vi "AguaClara Server Test.vi"() -> ()   [LabVIEW 2015, in "AguaClara Library.lvlib"]
uses:
  AguaClara Library.lvlib
  mathcad/Simple/MathCAD cmd.ctl
  <vilib>/Utility/SMTP/NI_SMTPEmail.lvlib
  Word cmd.ctl
  Variable cluster.ctl
  User Information.ctl
  Project inputs.ctl
  Basic Inputs.ctl
  user project design.ctl
  ADT Commands.ctl
  Country Ring.ctl
panel:
  in  "reload MathCAD":bool
  out "total requests":i32
  in  "ADT version":i32
  out "Revision":i32
  in  "SVN Checkout":bool
  in  "Progress bar":dbl(slide) max=314.0 scale=0.0..1.0
  out "DesignLog":refnum<file>
  out "Designs in queue":i32
  out "Loaded CAD":bool
  in  "File Directories":bool
  in  "millisecond multiple":u32=100
  out "stop loops":bool
  in  "stop":bool
  in  "Tab Control":T1(tab)=enum."Test Design"
  out "User Project Design":T2[](array[typedef])
  out "MathCAD Results":T3
  out "Find-Replace":cluster{"Find":string, "Replace":string}[](array[cluster])
  in  "Load Client Design":i32
  in  "Design Inputs":T4={"Q.Plant"=0.005, "C.CoagDoseMax"=0.1, "C.CoagStock"=120.0, "Ti.CoagStock"=108000.0, "EN.DrillSeries"=enum."English", "EN.TubeSeries"=enum."English", "N.SedTanks"=8.0, "N.SedBaysEst"=2.0, "W.SedPlate"=0.01, "L.SedPlateSheet"=1.08, "T.SedPlate"=3.0, "T.PlantWall"=0.002, "H.FlocOption"=0.15, "T.FlocBaffleRigidH"=1.0, "T.ConcreteMin"=0.04, "T.SedWeir"=0.05, "T.FlocBaffleRigidV"=0.05} caption="Basic Inputs" {"T.FlocBaffleRigidV" min=0.0 max=0.2 step=0.001 format="%#.1f"; "T.SedWeir" min=0.001 max=0.2 step=0.001 format="%#.1f"; "T.SedPlate" min=0.001 max=0.05 step=0.001 format="%#.1f"; "T.FlocBaffleRigidH" min=0.0 max=0.2 step=0.001 format="%#.1f"; "T.ConcreteMin" min=0.005 max=0.2 step=0.001 format="%#.1f"; "L.SedPlateSheet" min=0.3 max=8.0 step=0.01 format="%#.1f"; "N.SedBaysEst" min=1.0 max=20.0 step=1.0 format="%#.0f"; "N.SedTanks" min=1.0 max=20.0 step=1.0 format="%#.0f"; "Ti.CoagStock" min=43200.0 max=360000.0 step=3600.0 format="%#.1f"; "H.FlocOption" min=0.5 max=4.0 step=0.01 format="%#.2f"; "C.CoagStock" min=50.0 max=500.0 step=1.0 format="%#.0f"; "C.CoagDoseMax" min=0.03 max=0.2 step=0.005 format="%#.0f"; "Q.Plant" min=0.001 max=0.2 step=0.0001 format="%#.1f"; "T.PlantWall" min=0.05 max=0.5 step=0.001 format="%#.1f"; "W.SedPlate" min=0.5 max=3.0 step=0.001 format="%#.1f"}
  in  "Project Info":T5={"Project Name"="ADT Server Test", "City"="Ithaca", "State"="NY", "Notes"="USA"} caption="Project Information"
  in  "User Information":T6={"First Name"="Agua", "Last Name"="Clara", "Email Address"="cuaguaclara@gmail.com", "Organization"="Cornell University", "Language"=enum."English", "Country"=0} {"Country" items=["Afghanistan", "Aland Islands", "Albania", "Algeria", "American Samoa", "Andorra", "Angola", "Anguilla", "Antarctica", "Antigua And Barbuda", "Argentina", "Armenia", "Aruba", "Australia", "Austria", "Azerbaijan", "Bahamas", "Bahrain", "Bangladesh", "Barbados", "Belarus", "Belgium", "Belize", "Benin", "Bermuda", "Bhutan", "Bolivia", "Bosnia And Herzegovina", "Botswana", "Bouvet Island", "Brazil", "British Indian Ocean Territory", "Brunei Darussalam", "Bulgaria", "Burkina Faso", "Burundi", "Cambodia", "Cameroon", "Canada", "Cape Verde", "Cayman Islands", "Central African Republic", "Chad", "Chile", "China", "Christmas Island", "Cocos (Keeling) Islands", "Colombia", "Comoros", "Congo", "Congo, The Democratic Republic Of The", "Cook Islands", "Costa Rica", "Cote D'Ivoire", "Croatia", "Cuba", "Cyprus", "Czech Republic", "Denmark", "Djibouti", "Dominica", "Dominican Republic", "Ecuador", "Egypt", "El Salvador", "Equatorial Guinea", "Eritrea", "Estonia", "Ethiopia", "Falkland Islands (Malvinas)", "Faroe Islands", "Fiji", "Finland", "France", "French Guiana", "French Polynesia", "French Southern Territories", "Gabon", "Gambia", "Georgia", "Germany", "Ghana", "Gibraltar", "Greece", "Greenland", "Grenada", "Guadeloupe", "Guam", "Guatemala", "Guernsey", "Guinea", "Guinea-Bissau", "Guyana", "Haiti", "Heard Island And Mcdonald Islands", "Holy See (Vatican City State)", "Honduras", "Hong Kong", "Hungary", "Iceland", "India", "Indonesia", "Iran, Islamic Republic Of", "Iraq", "Ireland", "Isle Of Man", "Israel", "Italy", "Jamaica", "Japan", "Jersey", "Jordan", "Kazakhstan", "Kenya", "Kiribati", "Korea, Democratic People'S Republic Of", "Korea, Republic Of", "Kuwait", "Kyrgyzstan", "Lao People'S Democratic Republic", "Latvia", "Lebanon", "Lesotho", "Liberia", "Libyan Arab Jamahiriya", "Liechtenstein", "Lithuania", "Luxembourg", "Macao", "Macedonia, The Former Yugoslav Republic Of", "Madagascar", "Malawi", "Malaysia", "Maldives", "Mali", "Malta", "Marshall Islands", "Martinique", "Mauritania", "Mauritius", "Mayotte", "Mexico", "Micronesia, Federated States Of", "Moldova, Republic Of", "Monaco", "Mongolia", "Montserrat", "Morocco", "Mozambique", "Myanmar", "Namibia", "Nauru", "Nepal", "Netherlands", "Netherlands Antilles", "New Caledonia", "New Zealand", "Nicaragua", "Niger", "Nigeria", "Niue", "Norfolk Island", "Northern Mariana Islands", "Norway", "Oman", "Pakistan", "Palau", "Palestinian Territory, Occupied", "Panama", "Papua New Guinea", "Paraguay", "Peru", "Philippines", "Pitcairn", "Poland", "Portugal", "Puerto Rico", "Qatar", "Reunion", "Romania", "Russian Federation", "Rwanda", "Saint Helena", "Saint Kitts And Nevis", "Saint Lucia", "Saint Pierre And Miquelon", "Saint Vincent And The Grenadines", "Samoa", "San Marino", "Sao Tome And Principe", "Saudi Arabia", "Senegal", "Serbia And Montenegro", "Seychelles", "Sierra Leone", "Singapore", "Slovakia", "Slovenia", "Solomon Islands", "Somalia", "South Africa", "South Georgia And The South Sandwich Islands", "Spain", "Sri Lanka", "Sudan", "Suriname", "Svalbard And Jan Mayen", "Swaziland", "Sweden", "Switzerland", "Syrian Arab Republic", "Taiwan, Province Of China", "Tajikistan", "Tanzania, United Republic Of", "Thailand", "Timor-Leste", "Togo", "Tokelau", "Tonga", "Trinidad And Tobago", "Tunisia", "Turkey", "Turkmenistan", "Turks And Caicos Islands", "Tuvalu", "Uganda", "Ukraine", "United Arab Emirates", "United Kingdom", "United States", "United States Minor Outlying Islands", "Uruguay", "Uzbekistan", "Vanuatu", "Venezuela", "Viet Nam", "Virgin Islands, British", "Virgin Islands, U.S.", "Wallis And Futuna", "Western Sahara", "Yemen", "Zambia", "Zimbabwe", "(Not Specified)"]}
  in  "Recreate Design":bool
  out "Date":string
  out "Last Design":i32
  out "init errors":errorcluster caption="error out"
  out "commandline":string
  out "SVN Checkout output":string
  out "design errors":errorcluster
  out "error out design log":errorcluster
  out "ADT Commands":T8
  out "ADT version client request":i32
  out "Successful Checkout":bool
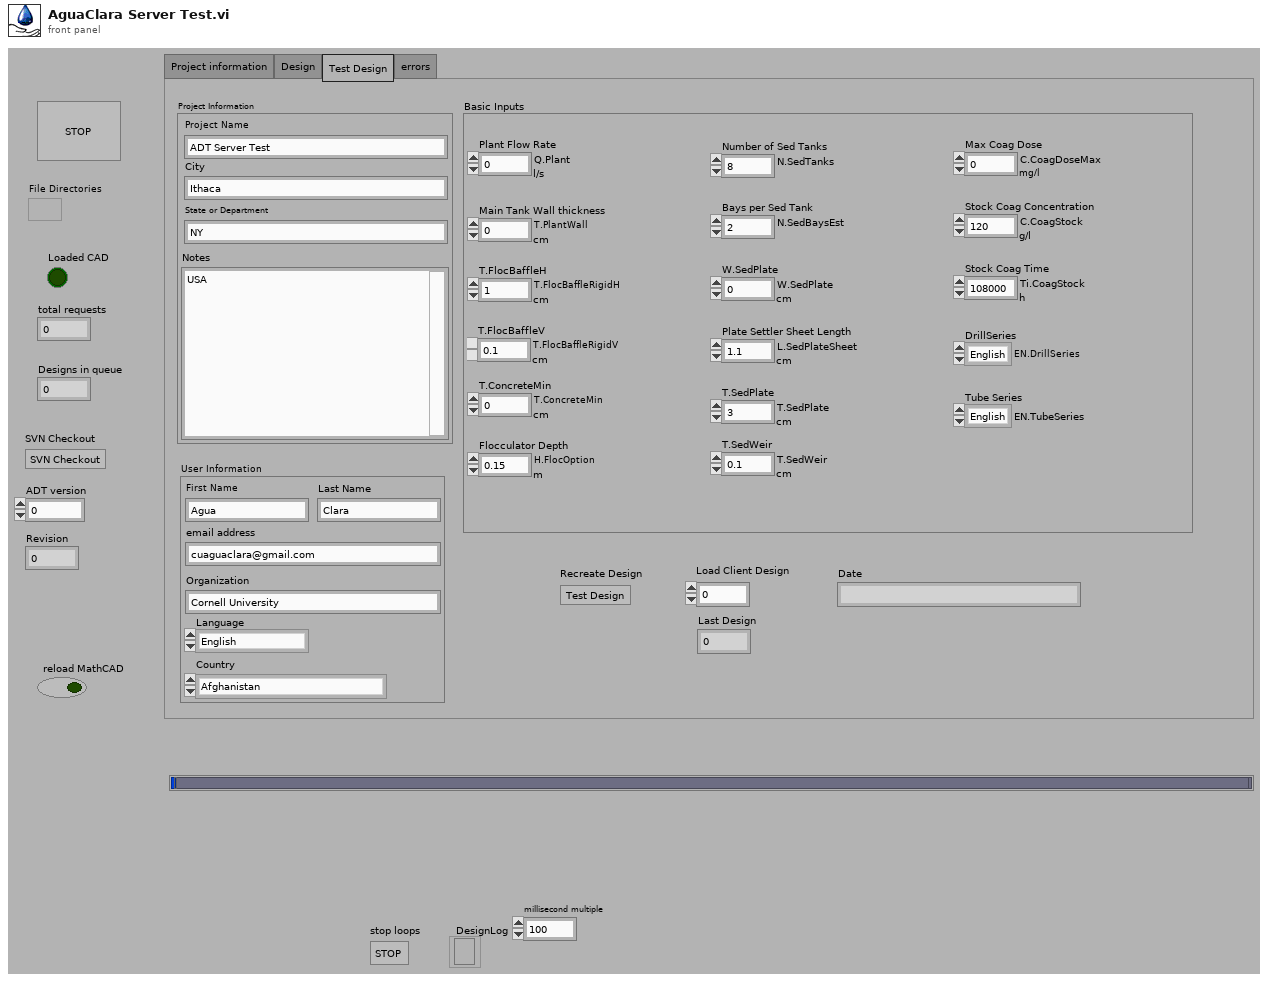
[diagram p1: front panel]
types:
  T1 = enum32{"Project information", "Design", "Test Design", "errors"}
  T2 = typedef "user project design.ctl" = cluster{"Key":string[], "Value":string[]}
  T3 = typedef "Variable cluster.ctl" = cluster{"Label.Text":string, "Control Type":u32, "Numeric":dbl, "Array":dbl[], "status":bool, "Str Array":string[], "String":string, "unit":string}[]
  T4 = typedef "AguaClara Library.lvlib/Basic Inputs.ctl" = cluster{"Q.Plant":dbl[unit], "C.CoagDoseMax":dbl[unit], "C.CoagStock":dbl[unit], "Ti.CoagStock":dbl[unit], "EN.DrillSeries":enum16{"English", "Metric"}, "EN.TubeSeries":enum16{"English", "Metric"}, "N.SedTanks":dbl, "N.SedBaysEst":dbl, "W.SedPlate":dbl[unit], "L.SedPlateSheet":dbl[unit], "T.SedPlate":dbl[unit], "T.PlantWall":dbl[unit], "H.FlocOption":dbl[unit], "T.FlocBaffleRigidH":dbl[unit], "T.ConcreteMin":dbl[unit], "T.SedWeir":dbl[unit], "T.FlocBaffleRigidV":dbl[unit]}
  T5 = typedef "AguaClara Library.lvlib/Project inputs.ctl" = cluster{"Project Name":string, "City":string, "State":string, "Notes":string}
  T6 = typedef "AguaClara Library.lvlib/User Information.ctl" = cluster{"First Name":string, "Last Name":string, "Email Address":string, "Organization":string, "Language":enum16{"English", "Español", "French"}, "Country":T7}
  T7 = typedef "Country Ring.ctl" = u16
  T8 = typedef "ADT Commands.ctl" = enum16{"Design Plant", "CheckOut MathCAD Files", "Restart"}
  T9 = enum16{"open", "replace", "create", "open or create", "replace or create", "replace or create with confirmation"}
  T10 = typedef "AguaClara Library.lvlib/Word cmd.ctl" = enum16{"Initialize", "Load User Inputs", "Update Fields", "Replace Variables", "Save pdf", "Close Word"}
  T11 = typedef "MathCAD cmd.ctl" = enum16{"Open App", "Open Worksheet", "Close Worksheet", "Load Variable Ref", "Send Number", "Send Cluster", "Send Array", "Send String", "Calculate", "Get MathCAD data", "Close MathCAD"}
  T12 = typedef "packed var.ctl" = variant
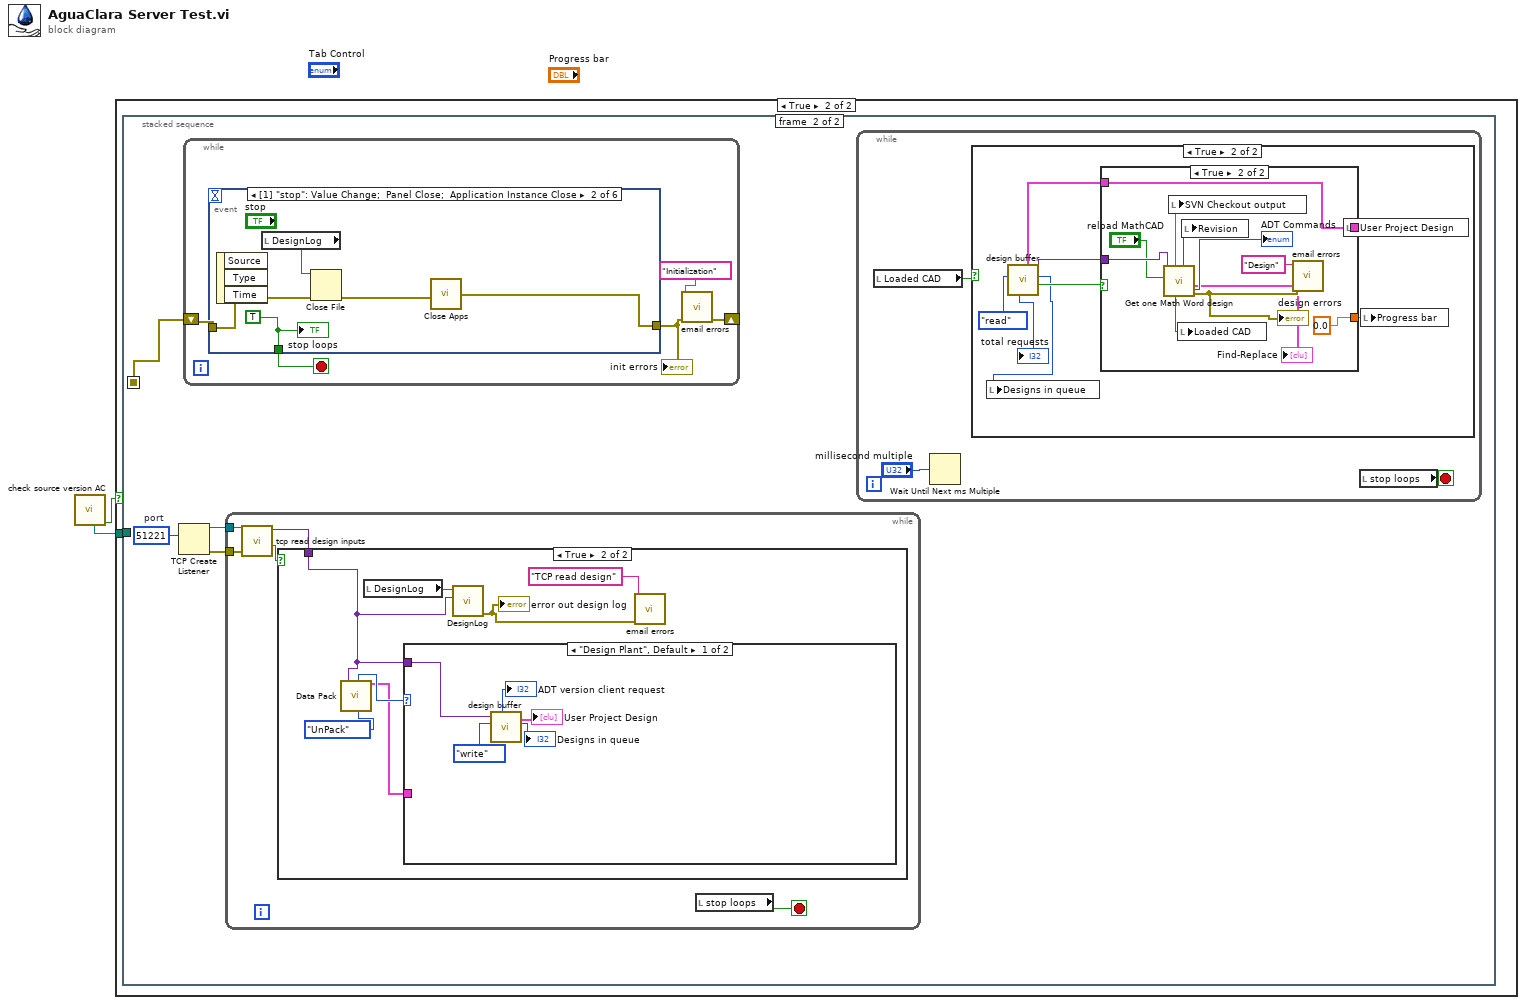
[diagram p0: block diagram]
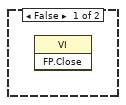
[diagram p2: hidden frame]
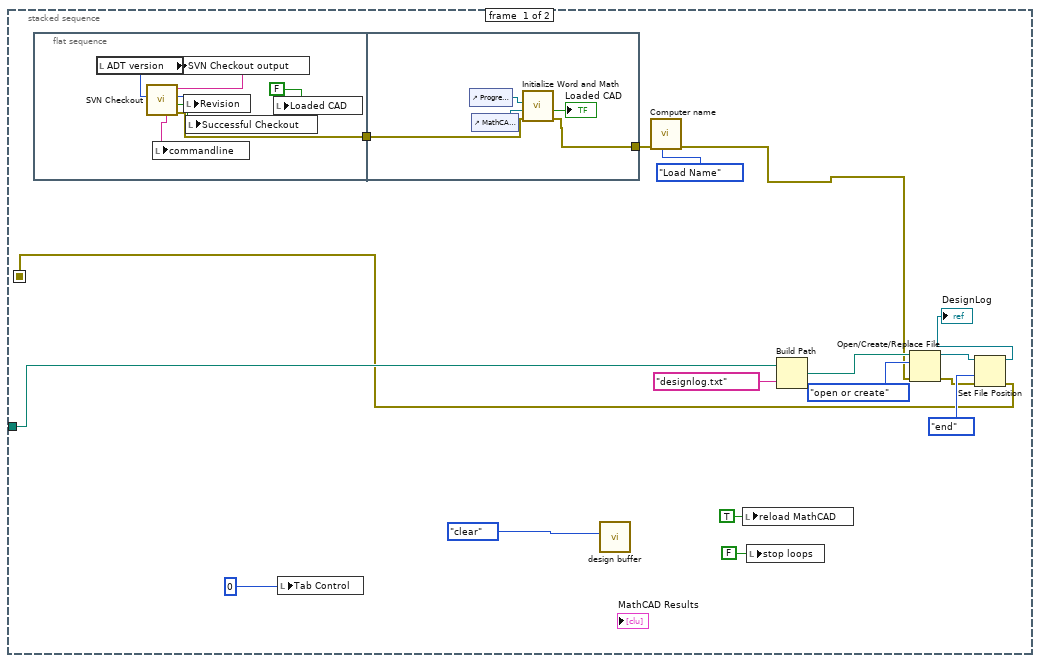
[diagram p3: hidden frame]
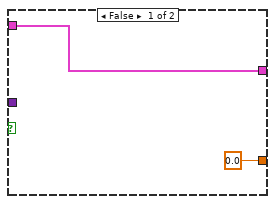
[diagram p5: hidden frame]
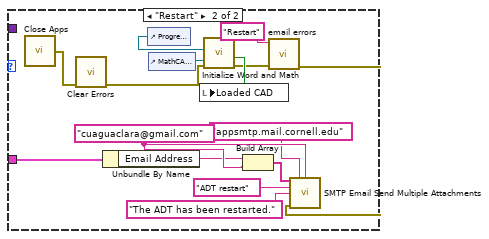
[diagram p7: hidden frame]
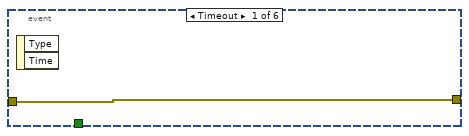
[diagram p8: hidden frame]
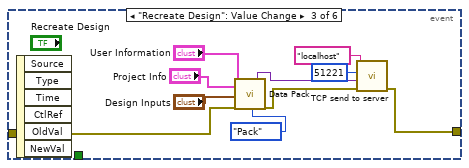
[diagram p9: hidden frame]
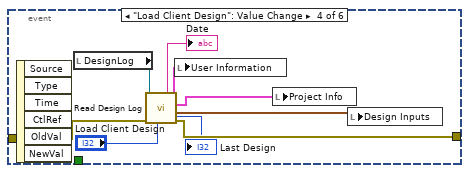
[diagram p10: hidden frame]
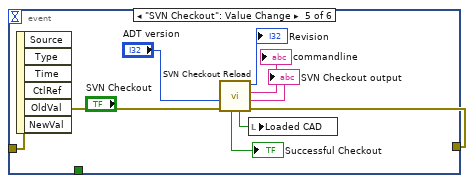
[diagram p11: hidden frame]
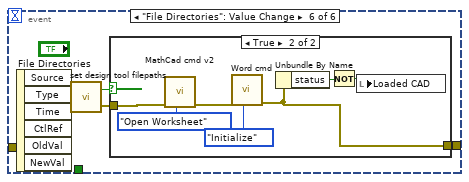
[diagram p12: hidden frame]
diagram:
  n1 = call "check source version AC.vi"() -> ("continue running?"=w2:bool, "Application folder"=w1:path)  [unwired: 3 in, 7 out]
  n2 = case shown="True" w2 {
    tunnel: w1 -> [_ w3]
    frame False {
      n3 = invoke class="VI" method="FP.Close"() -> ()  [unwired: 3 in, 3 out]
    }
    frame True {
      n4 = stacked-sequence {
        seq-local: [w9 _] -> [_ w36]
        tunnel: w3 -> [w14 _]
        frame #0 {
          n5 = flat-sequence {
            tunnel: [w23] -> w5
            tunnel: [w32] -> w7
            tunnel: w5 -> [w31]
            frame #0 {
              n6 = local read "ADT version"() -> (w26:i32)
              n7 = call "SVN Checkout.vi"("ADT version"=w26) -> ("error out"=w23:errorcluster, "Successful Checkout"=w21:bool, "Revision"=w24:i32, "standard output"=w25:string, "commandline"=w22:string)  [unwired: 6 in]
              n8 = local write "commandline"(w22) -> ()
              n9 = local write "SVN Checkout output"(w25) -> ()
              n10 = local write "Revision"(w24) -> ()
              n11 = local write "Successful Checkout"(w21) -> ()
              n12 = local write "Loaded CAD"(FALSE ("Loaded CAD")) -> ()
            }
            frame #1 {
              n13 = control-ref of="Progress bar"() -> (w29:refnum<vi>)
              n14 = control-ref of="MathCAD Results"() -> (w30:refnum<vi>)
              n15 = call "Initialize Word and Math.vi"("error in (no error)"=w31, "MathCAD results"=w30, "Slide Refnum"=w29) -> ("error out"=w32:errorcluster, "Success"=→"Loaded CAD":bool)  [unwired: 7 in]
            }
          }
          n16 = local write "Tab Control"(u8 0 ("Disabled")) -> ()
          n17 = call "design buffer.vi"("action"=enum16{"write", "read", "clear"}."clear") -> ()  [unwired: 3 in, 8 out]
          n18 = call "Computer name.vi"("cmd"=enum16{"Load Name", "Read Name"}."Load Name", "error in (no error)"=w7) -> ("error out"=w4:errorcluster)  [unwired: 8 in, 1 out]
          n19 = local write "reload MathCAD"(TRUE ("reload MathCAD")) -> ()
          n20 = local write "stop loops"(FALSE ("stop loops")) -> ()
          n21 = Build Path(base path=w14, name or relative path="designlog.txt") -> (appended path=w16:path)
          n22 = Open/Create/Replace File(file path (use dialog)=w16, error in=w4, operation (0:open)=T9."open or create") -> (refnum out=w11:refnum<file>, error out=w12:errorcluster)  [unwired: 3 in, 1 out]
          n23 = Set File Position(refnum=w11, from (0:start)=enum16{"start", "end", "current"}."end", error in=w12) -> (refnum out=→"DesignLog":refnum<file>, error out=w9:errorcluster)  [unwired: 1 in]
        }
        frame #1 {
          w35 = u16 51221  # port
          n24 = TCP Create Listener(10:w35) -> (0:w34:errorcluster, 3:w33:refnum<k5>)  [unwired: 4 in, 1 out]
          n25 = while {
            shift-right: [w95] -> _
            shift-left: w36 -> [w96]
            stop <- w97 stop-if-true
            n26 = event shown="[1] \"stop\": Value Change;  Panel Close;  Application Instance Close" {
              selector: _ -> [_ _ _ _ _ _]
              dyn-events: _ -> [_ _ _ _ _ _]
              timeout: _ -> [_ _ _ _ _ _]
              tunnel: [_ w101 _ _ _ _] -> w97
              tunnel: [w98 w99 w105 w121 w129 w132] -> w94
              tunnel: w96 -> [w98 w102 w106 w122 w130 _]
              event Timeout {
                n27 = event-data() -> ()  [unwired: 1 in, 2 out]
              }
              event "stop": Value Change; Panel Close; Application Instance Close {
                w101 = TRUE
                n28 = event-data() -> ()  [unwired: 1 in, 3 out]
                n29 = local read "DesignLog"() -> (w103:refnum<file>)
                n30 = Close File(refnum=w103, error in=w102) -> (error out=w100:errorcluster)  [unwired: 1 out]
                n31 = call "Close Apps.vi"("error in"=w100) -> ("error out"=w99:errorcluster)
                "stop loops" <- w101
              }
              event "Recreate Design": Value Change {
                n32 = event-data() -> ()  [unwired: 1 in, 6 out]
                n33 = call "Data Pack.vi"("User Information"="User Information", "Project Info"="Project Info", "Design Inputs"="Design Inputs", "error in"=w106, "Data transform"=enum16{"Pack", "UnPack"}."Pack") -> ("Packed Out"=w109:T12, "error out"=w107:errorcluster)  [unwired: 7 in, 6 out]
                n34 = call "TCP send to server.vi"("error in (no error)"=w107, "Packed In"=w109, "Port"=u16 51221, "Machine"="localhost") -> ("error out"=w105:errorcluster)  [unwired: 6 in, 1 out]
              }
              event "Load Client Design": Value Change {
                n35 = event-data() -> ()  [unwired: 1 in, 6 out]
                n36 = local read "DesignLog"() -> (w115:refnum<file>)
                n37 = call "Read Design Log.vi"("Design Log Index"="Load Client Design", "error in (no error)"=w122, "DesignLog"=w115) -> ("error out"=w121:errorcluster, "Design Inputs"=w118:T4, "Project inputs"=w119:T5, "User Information"=w117:T6, "Last Design"=→"Last Design":i32, "Date"=→"Date":string)  [unwired: 3 in]
                n38 = local write "User Information"(w117) -> ()
                n39 = local write "Project Info"(w119) -> ()
                n40 = local write "Design Inputs"(w118) -> ()
              }
              event "SVN Checkout": Value Change {
                n41 = event-data() -> ()  [unwired: 1 in, 6 out]
                n42 = call "SVN Checkout Reload.vi"("error in"=w130, "ADT version"="ADT version") -> ("error out"=w129:errorcluster, "SVN Checkout output"=→"SVN Checkout output":string, "commandline"=→"commandline":string, "Revision"=→"Revision":i32, "Success"=w125:bool, "Successful Checkout"=→"Successful Checkout":bool)  [unwired: 4 in]
                n43 = local write "Loaded CAD"(w125) -> ()
              }
              event "File Directories": Value Change {
                n44 = event-data() -> ()  [unwired: 1 in, 6 out]
                n45 = call "set design tool filepaths.vi"() -> ("error out"=w133:errorcluster, "Success"=w131:bool)  [unwired: 2 in]
                n46 = case shown="True" w131 {
                  tunnel: w133 -> [w134 w141]
                  tunnel: [w134 w135] -> w132
                  frame False {
                  }
                  frame True {
                    n47 = call "MathCad cmd v2.vi"("MathCAD cmds"=MathCAD_cmd."Open Worksheet", "error in"=w141) -> ("first error out"=w136:errorcluster)  [unwired: 8 in, 1 out]
                    n48 = call "Word cmd.vi"("Word cmd"=Word_cmd."Initialize", "Error In (no error)"=w136) -> ("error out"=w135:errorcluster)  [unwired: 8 in, 1 out]
                    n49 = Unbundle By Name(w135) -> ("status"=w139:bool)
                    n50 = Not(x=w139) -> (.not. x?=w138:bool)
                    n51 = local write "Loaded CAD"(w138) -> ()
                  }
                }
              }
            }
            "init errors" <- w94
            n52 = call "email errors.vi"("error in (no error)"=w94, "Loop id"="Initialization") -> ("error out (no error)"=w95:errorcluster)  [unwired: 9 in]
          }
          n53 = while {
            tunnel: w34 -> [w63]
            tunnel: w33 -> [w62]
            stop <- w65 stop-if-true
            n54 = call "tcp read design inputs.vi"("error in (no error)"=w63, "listener ID in"=w62) -> ("success"=w61:bool, "Design Inputs"=w64:variant)  [unwired: 7 in, 1 out]
            n55 = case shown="True" w61 {
              tunnel: w64 -> [_ w69]
              frame False {
              }
              frame True {
                n56 = call "Data Pack.vi"("Packed In"=w69, "Data transform"=enum16{"Pack", "UnPack"}."UnPack") -> ("ADT Commands out"=w67:T8, "User Information out"=w66:T6)  [unwired: 10 in, 6 out]
                n57 = local read "DesignLog"() -> (w72:refnum<file>)
                n58 = case shown="\"Design Plant\", Default" w67 {
                  tunnel: w69 -> [w77 _]
                  tunnel: w66 -> [_ w81]
                  frame "Design Plant", Default {
                    n59 = call "design buffer.vi"("action"=enum16{"write", "read", "clear"}."write", "Design Inputs"=w77) -> ("buffer size"=→"Designs in queue":i32, "User Project Design"=→"User Project Design":T2[], "ADT Version"=→"ADT version client request":i32)  [unwired: 2 in, 5 out]
                  }
                  frame "Restart" {
                    w84 = "cuaguaclara@gmail.com" ("return address")
                    n60 = call "Close Apps.vi"() -> ("error out"=w79:errorcluster)  [unwired: 1 in]
                    n61 = call <vilib>:"Clear Errors.vi"("error in (no error)"=w79) -> ("error out"=w78:errorcluster)  [unwired: 5 in, 1 out]
                    n62 = Unbundle By Name(w81) -> ("Email Address"=w83:string)
                    n63 = control-ref of="Progress bar"() -> (w91:refnum<vi>)
                    n64 = control-ref of="MathCAD Results"() -> (w92:refnum<vi>)
                    n65 = call "Initialize Word and Math.vi"("error in (no error)"=w78, "MathCAD results"=w92, "Slide Refnum"=w91) -> ("error out"=w89:errorcluster, "Success"=w90:bool)  [unwired: 7 in]
                    n66 = local write "Loaded CAD"(w90) -> ()
                    n67 = Build Array(w83, w84) -> (w85:string[])
                    n68 = call "email errors.vi"("error in (no error)"=w89, "Loop id"="Restart") -> ("error out (no error)"=w80:errorcluster)  [unwired: 9 in]
                    n69 = call <vilib>:"SMTP Email Send Multiple Attachments.vi"("recipients"=w85, "mail server"="appsmtp.mail.cornell.edu", "return address"=w84, "subject ([No Subject])"="ADT restart", "message"="The ADT has been restarted." ("subject ([No Subject])"), "error in (no error)"=w80) -> ()  [unwired: 8 in, 2 out]
                  }
                }
                n70 = call "DesignLog.vi"("variant"=w69, "DesignLog"=w72) -> ("error out"=w70:errorcluster)  [unwired: 8 in, 1 out]
                "error out design log" <- w70
                n71 = call "email errors.vi"("error in (no error)"=w70, "Loop id"="TCP read design") -> ()  [unwired: 9 in, 1 out]
              }
            }
            n72 = local read "stop loops"() -> (w65:bool)
          }
          n73 = while {
            stop <- w39 stop-if-true
            n74 = local read "Loaded CAD"() -> (w38:bool)
            n75 = Wait Until Next ms Multiple(millisecond multiple="millisecond multiple") -> ()  [unwired: 1 out]
            n76 = case shown="True" w38 {
              frame False {
              }
              frame True {
                n77 = call "design buffer.vi"("action"=enum16{"write", "read", "clear"}."read") -> ("got data"=w45:bool, "buffer size"=w44:i32, "Design Inputs Out"=w46:T12, "User Project Design"=w42:T2[], "writes"=→"total requests":i32)  [unwired: 3 in, 3 out]
                n78 = local write "Designs in queue"(w44) -> ()
                n79 = case shown="True" w45 {
                  tunnel: w46 -> [_ w60]
                  tunnel: w42 -> [w49 w56]
                  tunnel: [w49 w56] -> w41
                  tunnel: [0.0 ("Progress bar") 0.0 ("Progress bar")] -> w40
                  frame False {
                  }
                  frame True {
                    n80 = call "Get one Math Word design.vi"("reload MathCAD"="reload MathCAD", "Design Inputs"=w60) -> ("error out"=w54:errorcluster, "ADT Commands"=→"ADT Commands":T8, "Revision"=w59:i32, "Success"=w58:bool, "SVN Checkout output"=w57:string, "Find-Replace"=→"Find-Replace":cluster{"Find":string, "Replace":string}[])  [unwired: 1 in, 3 out]
                    "design errors" <- w54
                    n81 = local write "SVN Checkout output"(w57) -> ()
                    n82 = local write "Loaded CAD"(w58) -> ()
                    n83 = local write "Revision"(w59) -> ()
                    n84 = call "email errors.vi"("error in (no error)"=w54, "Loop id"="Design") -> ()  [unwired: 9 in, 1 out]
                  }
                }
                n85 = local write "User Project Design"(w41) -> ()
                n86 = local write "Progress bar"(w40) -> ()
              }
            }
            n87 = local read "stop loops"() -> (w39:bool)
          }
        }
      }
    }
  }
